vi "task_3.vi"() -> ()   [LabVIEW 2020]
panel:
  in  "White":bool
  out "White LED":bool
  out "Count":i32
  out "Top 3":cluster{"Player1":string, "Score":i32}[](array[cluster])
  out "Player Info":cluster{"Player1":string, "Score":i32}
  in  "Blue":bool
  out "Blue LED":bool
  in  "Red":bool
  out "Red LED":bool
  in  "Green":bool
  out "Green LED":bool
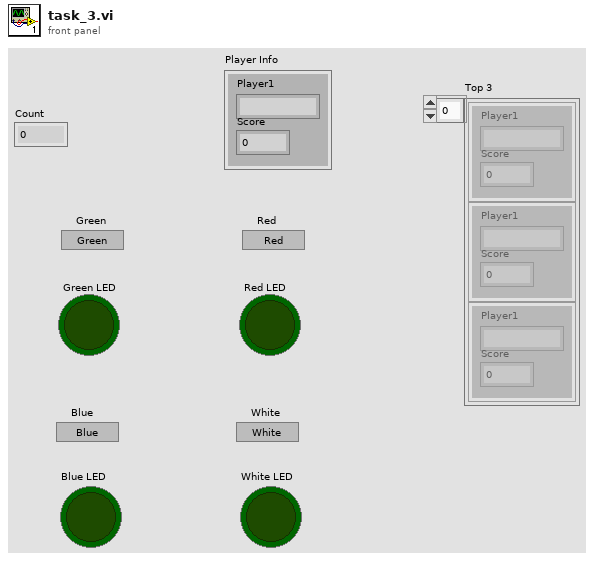
[diagram p1: front panel]
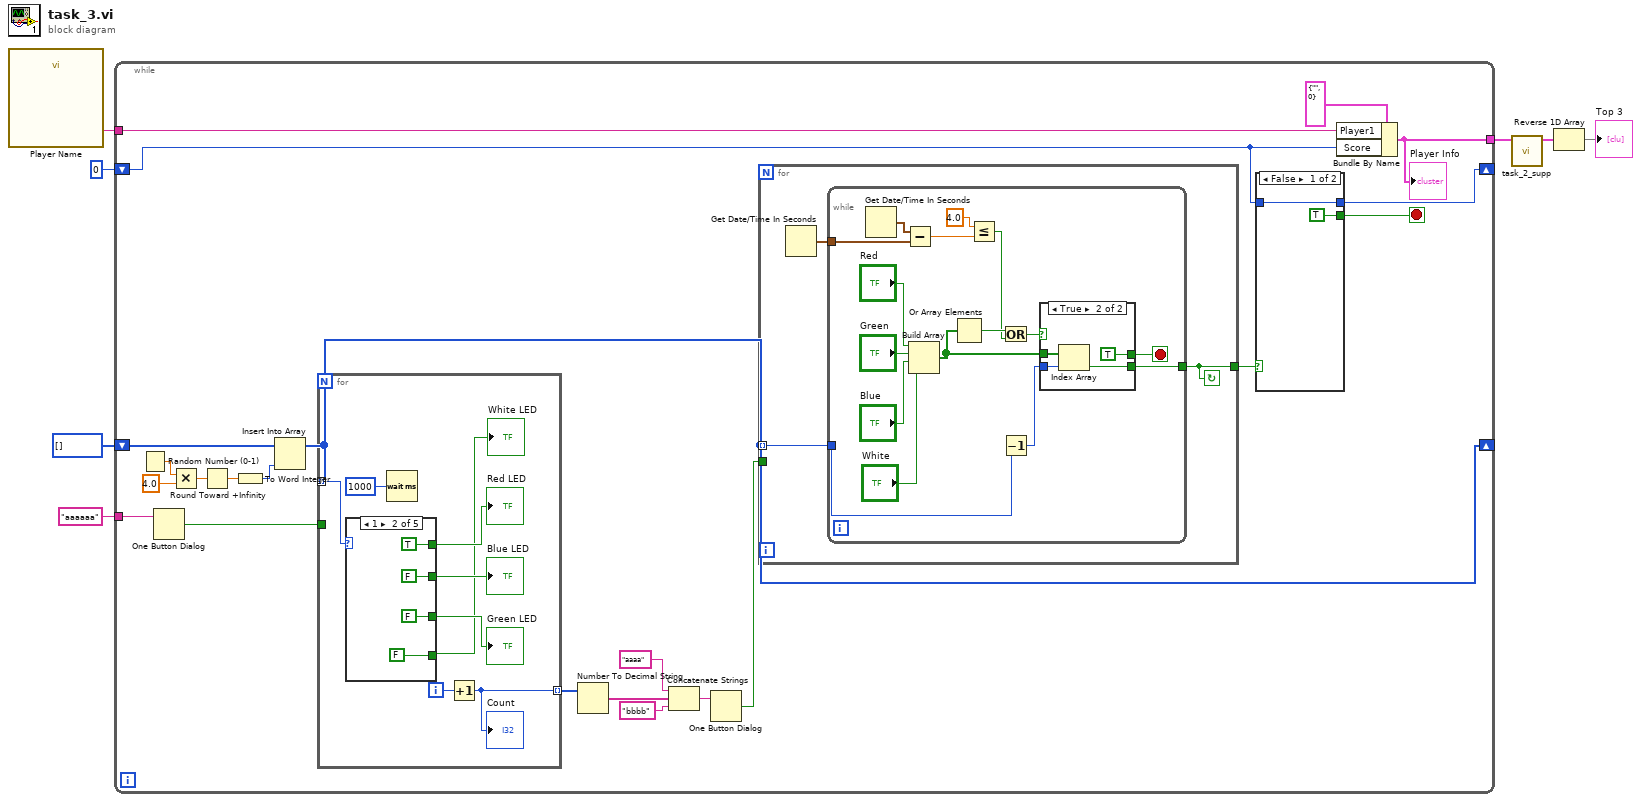
[diagram p0: block diagram]
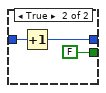
[diagram p2: hidden frame]
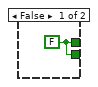
[diagram p3: hidden frame]
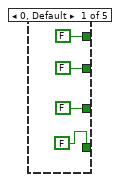
[diagram p4: hidden frame]
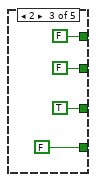
[diagram p5: hidden frame]
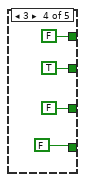
[diagram p6: hidden frame]
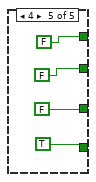
[diagram p7: hidden frame]
diagram:
  n1 = call "Player Name"() -> ("name"=w4:string)  [unwired: 17 in, 2 out]
  n2 = while {
    tunnel: [w25] -> w5
    tunnel: w4 -> [w24]
    shift-right: [w22] -> _
    shift-left: 0 -> [w23]
    tunnel: "aaaaaa" -> [w21]
    shift-right: [w11] -> _
    shift-left: i32[] [] -> [w18]
    stop <- w9 stop-if-true
    n3 = Random Number (0-1)() -> (number: 0 to 1=w29:dbl)
    n4 = One Button Dialog(message=w21) -> (true=w20:bool)  [unwired: 1 in]
    n5 = Multiply(x=w29, y=4.0) -> (x*y=w28:dbl)
    n6 = Round Toward +Infinity(x=w28) -> (ceil(x): smallest int >= x=w27:dbl)
    n7 = To Word Integer(number=w27) -> (16bit integer=w19:i16)
    n8 = Insert Into Array(array=w18, new element=w19) -> (w11:i32[])  [unwired: 1 in]
    n9 = for {
      tunnel: w20 -> [_]
      tunnel: w11 -> [w65] mode=indexing
      tunnel: [w60] -> w17 mode=indexing
      i -> [w61]
      n10 = case shown="1" w65 {
        tunnel: [FALSE TRUE FALSE FALSE FALSE] -> w64
        tunnel: [FALSE FALSE TRUE FALSE FALSE] -> w63
        tunnel: [FALSE FALSE FALSE TRUE FALSE] -> w62
        tunnel: [FALSE FALSE FALSE FALSE TRUE] -> w59
        frame 0, Default {
        }
        frame 1 {
        }
        frame 2 {
        }
        frame 3 {
        }
        frame 4 {
        }
      }
      "Green LED" <- w63
      "Blue LED" <- w62
      "Red LED" <- w64
      "White LED" <- w59
      n11 = Wait (ms)(milliseconds to wait=1000) -> ()  [unwired: 1 out]
      n12 = Increment(x=w61) -> (x+1=w60:i32)
      "Count" <- w60
    }
    n13 = Number To Decimal String(number=w17) -> (decimal integer string=w16:string[])  [unwired: 1 in]
    n14 = Concatenate Strings("aaaa", w16, "bbbb") -> (w13:string)
    n15 = One Button Dialog(message=w13) -> (true=w12:bool)  [unwired: 1 in]
    n16 = for {
      tunnel: w12 -> [_]
      tunnel: w11 -> [w37] mode=indexing
      tunnel: [w35] -> w10
      stop <- w35 continue-if-true
      n17 = Get Date/Time In Seconds() -> (seconds since 1Jan1904=w36:timestamp)
      n18 = while {
        tunnel: w37 -> [w53]
        tunnel: [w43] -> w35
        tunnel: w36 -> [w48]
        stop <- w42 stop-if-true
        n19 = Get Date/Time In Seconds() -> (seconds since 1Jan1904=w49:timestamp)
        n20 = Subtract(x=w49, y=w48) -> (x-y=w41:dbl)
        n21 = Build Array("Red", "Green", "Blue", "White") -> (w46:bool[])
        n22 = Or Array Elements(Boolean array=w46) -> (logical OR=w45:bool)
        n23 = Less Or Equal?(x=4.0, y=w41) -> (x <= y?=w39:bool)
        n24 = Or(x=w45, y=w39) -> (x .or. y?=w44:bool)
        n25 = Decrement(x=w53) -> (x-1=w47:i32)
        n26 = case shown="True" w44 {
          tunnel: w46 -> [_ w58]
          tunnel: w47 -> [_ w57]
          tunnel: [w54 w56] -> w43
          tunnel: [w54 TRUE] -> w42
          frame False {
            w54 = FALSE
          }
          frame True {
            n27 = Index Array(array=w58, index=w57) -> (element=w56:bool)
          }
        }
      }
    }
    n28 = case shown="False" w10 {
      tunnel: w23 -> [w31 w34]
      tunnel: [w31 w33] -> w22
      tunnel: [TRUE FALSE] -> w9
      frame False {
      }
      frame True {
        n29 = Increment(x=w34) -> (x+1=w33:i32)
      }
    }
    n30 = Bundle By Name(cluster=cluster{"Player1":string, "Score":i32} {"Player1"="", "Score"=0} ("Player Info"), "Player1"=w24, "Score"=w23) -> (w25:cluster{"Player1":string, "Score":i32})
    "Player Info" <- w25
  }
  n31 = call "task_2_supp.vi"("Player Info"=w5) -> ("Array"=w7:cluster{"Player1":string, "Score":i32}[])  [unwired: 10 in]
  n32 = Reverse 1D Array(array=w7) -> (reversed array=→"Top 3":cluster{"Player1":string, "Score":i32}[])
